vi "libc path.vi"(8 "error in (no error)":errorcluster) -> (0 "error out":errorcluster, 3 "path to library":path)   [LabVIEW 2013, in "Linux Errno.lvlib"]
uses:
  Linux Errno.lvlib
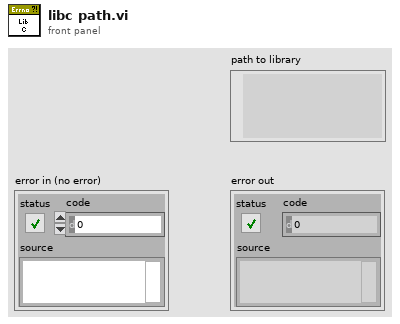
[diagram p1: front panel]
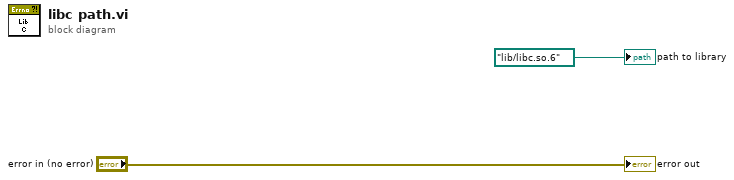
[diagram p0: block diagram]
diagram:
  "path to library" <- path "/lib/libc.so.6" ("path in")
  "error out" <- "error in (no error)"
